vi "6.vi"(11 "文字列入力":string) -> (3 "文字列出力":string)   [LabVIEW 2019]
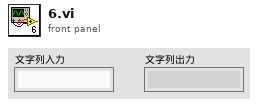
[diagram p1: front panel]
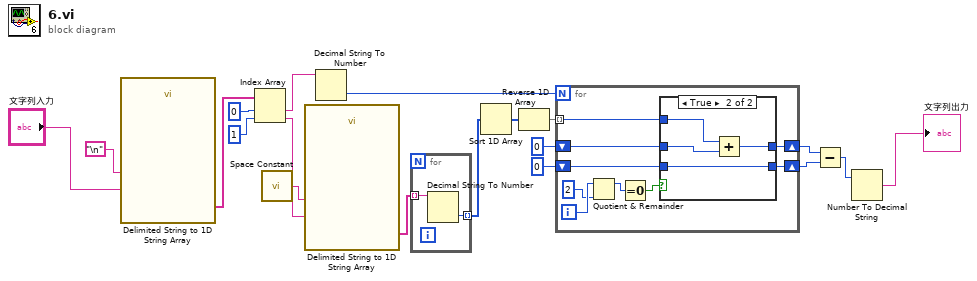
[diagram p0: block diagram]
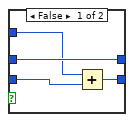
[diagram p2: hidden frame]
diagram:
  n1 = call <vilib>:"Delimited String to 1D String Array.vi"("delimiter"="\n", "delimited string"="文字列入力") -> ("string array"=w4:string[])  [unwired: 9 in]
  n2 = Index Array ("指標配列")(array=w4, index #1=0, index #2=1) -> (element #1=w8:string, element #2=w9:string)
  n3 = call <vilib>:"Space Constant.vi"() -> ("String"=w10:string)
  n4 = call <vilib>:"Delimited String to 1D String Array.vi"("delimiter"=w10, "delimited string"=w9) -> ("string array"=w11:string[])  [unwired: 9 in]
  n5 = Decimal String To Number(string=w8) -> (number=w12:i32)  [unwired: 2 in, 1 out]
  n6 = for {
    tunnel: w11 -> [w21] mode=indexing
    tunnel: [w20] -> w13 mode=indexing
    n7 = Decimal String To Number(string=w21) -> (number=w20:i32)  [unwired: 2 in, 1 out]
  }
  n8 = Sort 1D Array(array=w13) -> (sorted array=w14:i32[])
  n9 = Reverse 1D Array(array=w14) -> (reversed array=w3:i32[])
  n10 = for {
    N: w12 -> [_]
    tunnel: w3 -> [w23] mode=indexing
    shift-right: [w26] -> w17
    shift-left: 0 -> [w27]
    shift-right: [w24] -> w18
    shift-left: 0 -> [w25]
    i -> [w30]
    n11 = Quotient & Remainder(x=w30, y=2) -> (x-y*floor(x/y)=w29:i32)  [unwired: 1 out]
    n12 = Equal To 0?(x=w29) -> (x = 0?=w28:bool)
    n13 = case shown="TRUE" w28 {
      tunnel: w27 -> [w34 w38]
      tunnel: [w34 w36] -> w26
      tunnel: w25 -> [w33 w37]
      tunnel: [w32 w37] -> w24
      tunnel: w23 -> [w31 w35]
      frame False {
        n14 = Add(x=w31, y=w33) -> (x+y=w32:i32)
      }
      frame True {
        n15 = Add(x=w35, y=w38) -> (x+y=w36:i32)
      }
    }
  }
  n16 = Subtract(x=w17, y=w18) -> (x-y=w19:i32)
  n17 = Number To Decimal String(number=w19) -> (decimal integer string=→"文字列出力":string)  [unwired: 1 in]
